vi "FPGAoutput_fixed_375.vi"() -> ()   [LabVIEW 2013]
uses:
  <vilib>/Platform/TimedLoop/XDataNode/timing_clust.ctl
  <vilib>/Platform/TimedLoop/XDataNode/nitl_modes.ctl
  <vilib>/Platform/TimedLoop/XDataNode/wakeup.ctl
  <vilib>/rvi/Emulation/niFpgaSctlEmulationGetInTimedLoop.vi
  <vilib>/rvi/Emulation/niFpgaEmulationReportErrorSimple.vi
  <vilib>/rvi/Emulation/niFpgaGetClockAttributes.vi
  <vilib>/rvi/eio/common/nirviEmuTemplateMethod_errors.vi
  <vilib>/rvi/Emulation/niFpgaCriticalErrorInLSC.vi
  <vilib>/Platform/TimedLoop/XDataNode/XDataNode.xnode
  <vilib>/eio/EIONode/EIONode.xnode
  <vilib>/Platform/TimedLoop/XDataNode/XDNodeRunTimeDep.lvlib
panel:
  out "IO Module\\Trigger Input":bool
  in  "User Command Commit":bool
  in  "User Command":u8
  out "User Command Idle":bool
  out "User Command Status":u8
  in  "User Data 0":u8
  in  "User Data 1":u8
  out "PLL Locked":bool
  out "User Error":bool
  out "Configured?":bool
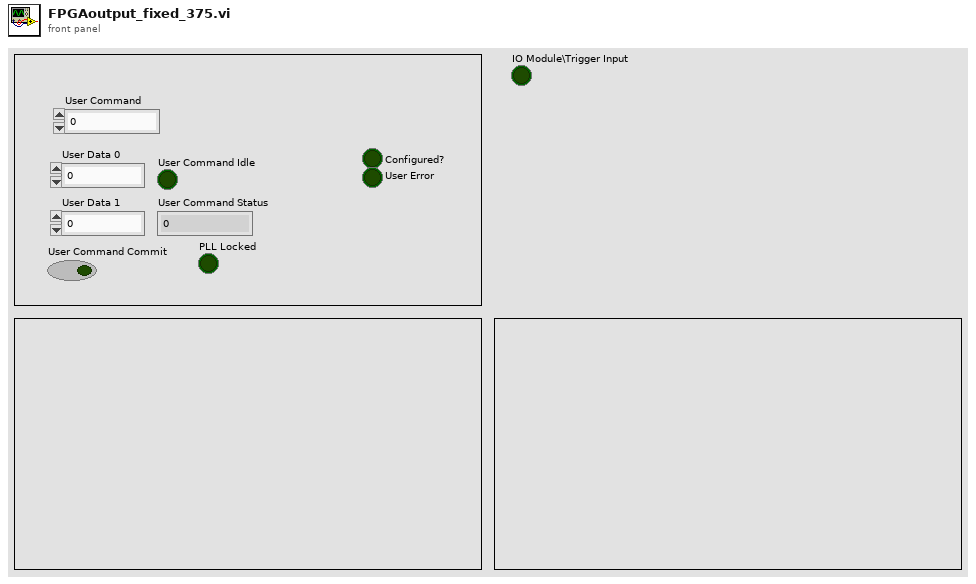
[diagram p1: front panel]
types:
  T1 = typedef "XDNodeRunTimeDep.lvlib/timing_clust.ctl" = cluster{"Expected End [f-1]":u64, "Actual End [f-1]":u64, "Finished Late? [f-1]":bool, "Expected End [i-1]":u64, "Actual End [i-1]":u64, "Finished Late? [i-1]":bool, "Expected Start [i]":u64, "Actual Start [i]":u64, "Expected Start [f]":u64, "Actual Start [f]":u64, "Source Name":string, "Structure Name":string, "Period":i64, "Deadline":i64, "Offset":i64, "Start":i64, "Priority":i32, "Timeout":i32, "Mode":T2, "Wakeup Reason":T3, "Error":errorcluster, "Source Type":string, "Secondary Source Type":string, "Global End Time":u64, "Global Start Time":u64, "Frame Duration":u64, "Iteration Duration":u64, "Assigned CPU":i32, "I/O Scan Engine Mode":u32}
  T2 = typedef "XDNodeRunTimeDep.lvlib/nitl_modes.ctl" = enum32{"No Change", "Process missed periods, maintain original phase", "Discard missed periods, maintain original phase", "Process missed periods, ignore original phase", "Discard missed periods, ignore original phase"}
  T3 = typedef "XDNodeRunTimeDep.lvlib/wakeup.ctl" = enum32{"Normal", "Aborted", "Asynchronous wakeup", "Timing source error", "Timed loop error", "Timeout"}
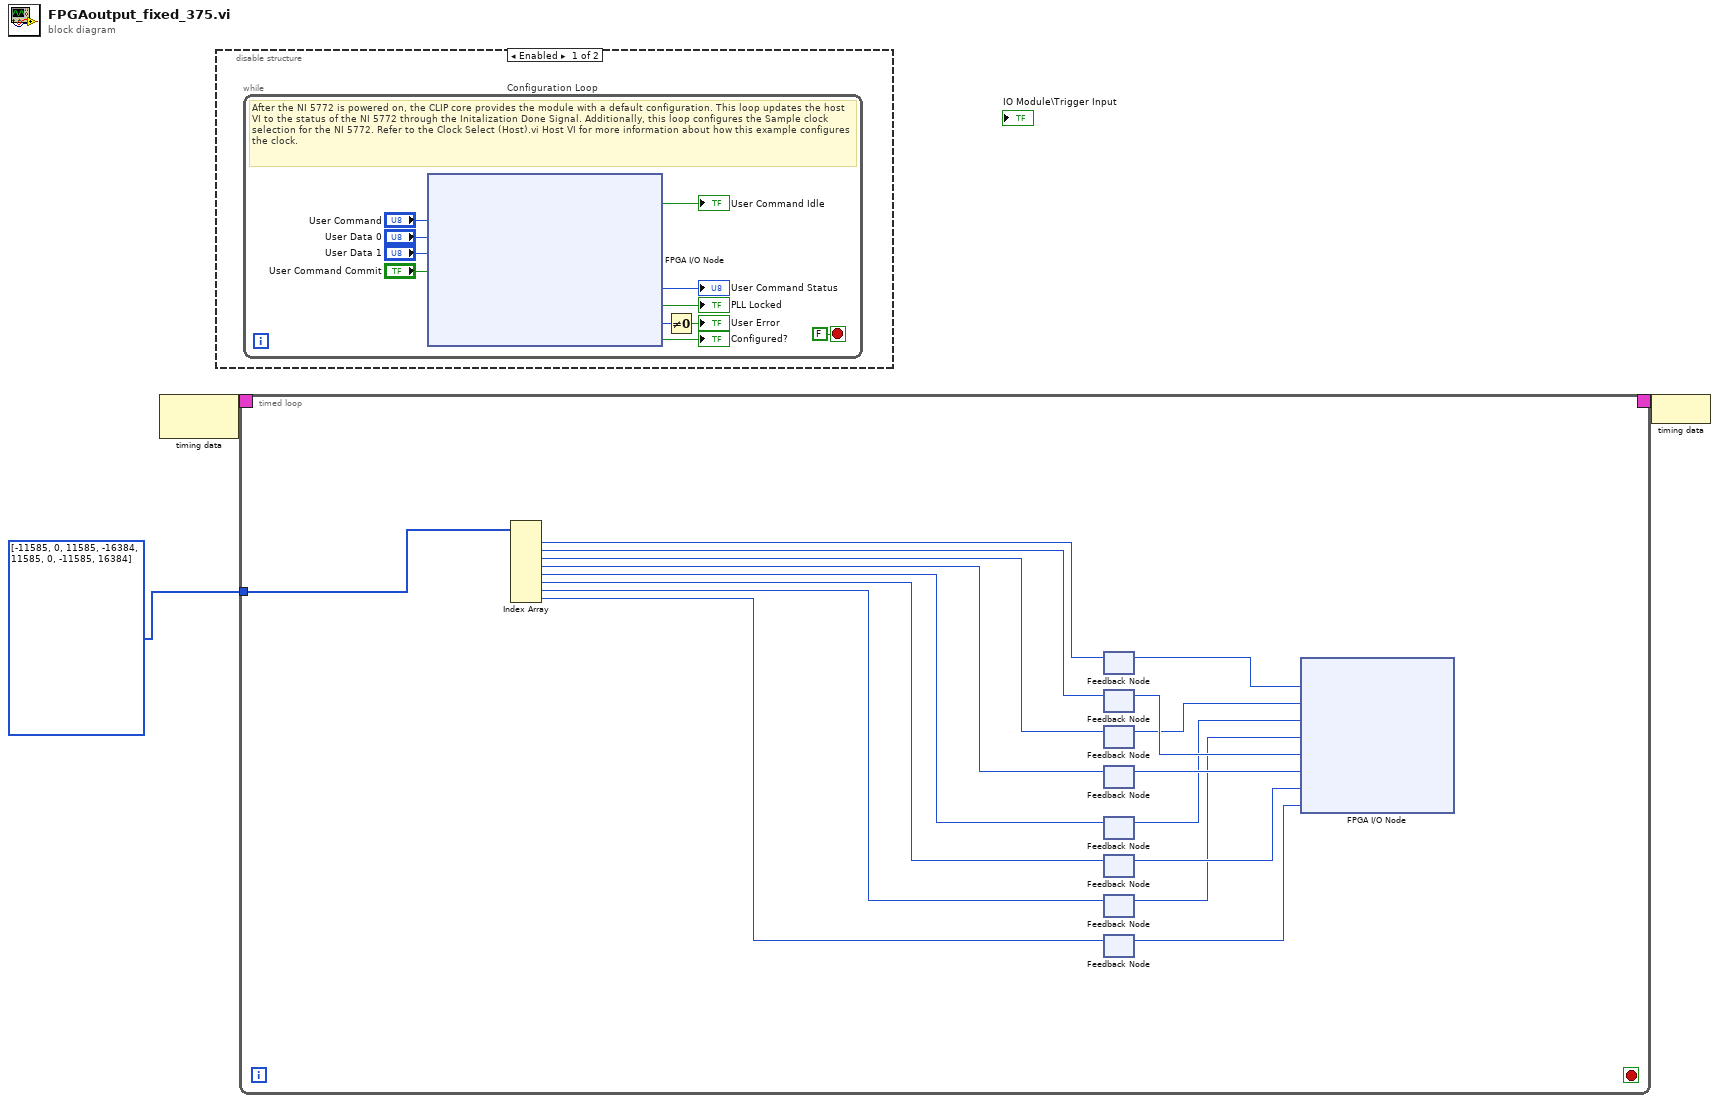
[diagram p0: block diagram]
diagram:
  n1 = node-c288() -> (w3:T1)  [unwired: 1 in]
  n2 = disable-structure shown="Enabled" {
    frame Enabled {
      n3 = while "Configuration Loop" {
        stop <- FALSE stop-if-true
        # "After the NI 5772 is powered on, the CLIP core provides the module with a default configuration. This loop updates the host VI to the status of the NI 5772 through the Initalization Done Signal. Additionally, this loop configures the Sample clock selection for the NI 5772. Refer to the Clock Select (Host).vi Host VI for more information about how this example configures the clock."
        n4 = xnode "FPGA I/O Node"("IO Module\\User Command"="User Command", "IO Module\\User Data 0"="User Data 0", "IO Module\\User Data 1"="User Data 1", "IO Module\\User Command Commit"="User Command Commit") -> ("IO Module\\User Command Idle"=→"User Command Idle":bool, "IO Module\\User Command Status"=→"User Command Status":u8, "IO Module\\PLL Locked"=→"PLL Locked":bool, "IO Module\\User Error"=w9:u8, "IO Module\\Initialization Done"=→"Configured?":bool)  [unwired: 9 in, 9 out]
        n5 = Not Equal To 0?(x=w9) -> (x != 0?=→"User Error":bool)
      }
    }
    frame Disabled {
    }
  }
  n6 = timed-loop {
    timing: w3 -> [_]
    timing-out: [_] -> w2
    tunnel: i16[] [-11585, 0, 11585, -16384, 11585, 0, -11585, 16384] ("output array 2") -> [w23]
    stop <- _ stop-if-true
    n7 = Index Array(array=w23) -> (element #1=w22:i16, element #2=w21:i16, element #3=w20:i16, element #4=w19:i16, element #5=w18:i16, element #6=w17:i16, element #7=w16:i16, element #8=w15:i16)  [unwired: 8 in]
    n8 = feedback #1() -> (w31:i16)  [unwired: 1 in]
    n9 = feedback-in #1(w22) -> ()
    n10 = feedback #2() -> (w30:i16)  [unwired: 1 in]
    n11 = feedback-in #2(w21) -> ()
    n12 = feedback #3() -> (w29:i16)  [unwired: 1 in]
    n13 = feedback-in #3(w20) -> ()
    n14 = feedback #4() -> (w28:i16)  [unwired: 1 in]
    n15 = feedback-in #4(w19) -> ()
    n16 = feedback #5() -> (w27:i16)  [unwired: 1 in]
    n17 = feedback-in #5(w18) -> ()
    n18 = feedback #6() -> (w26:i16)  [unwired: 1 in]
    n19 = feedback-in #6(w17) -> ()
    n20 = feedback #7() -> (w25:i16)  [unwired: 1 in]
    n21 = feedback-in #7(w16) -> ()
    n22 = feedback #8() -> (w24:i16)  [unwired: 1 in]
    n23 = feedback-in #8(w15) -> ()
    n24 = xnode "FPGA I/O Node"("IO Module\\AO 0 N-3"=w31, "IO Module\\AO 0 N-2"=w29, "IO Module\\AO 0 N-1"=w27, "IO Module\\AO 0 N"=w25, "IO Module\\AO 1 N-3"=w30, "IO Module\\AO 1 N-2"=w28, "IO Module\\AO 1 N-1"=w26, "IO Module\\AO 1 N"=w24) -> ()  [unwired: 8 in, 8 out]
  }
  n25 = node-c288(w2) -> ()
